vi "Configure 4Wire Resistance.vi"(0 "VISA resource name":refnum<visa-resource-name>, 1 "NPLC":u16(ring) items=["0.00005", "1", "12", "15"], 2 "Offset Compensation":bool, 5 "Auto Range? (T: Auto)":bool, 7 "Manual Range":dbl, 9 "Aperture Seconds":dbl, 11 "error in (no error)":errorcluster, 12 "Enable Dry Circuit":bool, 13 "Detection of Open Leads":bool) -> (4 "VISA resource name out":refnum<visa-resource-name>, 15 "error out":errorcluster)   [LabVIEW 2009, in "Keithley DMM7510.lvlib"]
doc: "This VI configures the 4 wire Resistance."
uses:
  Keithley DMM7510.lvlib
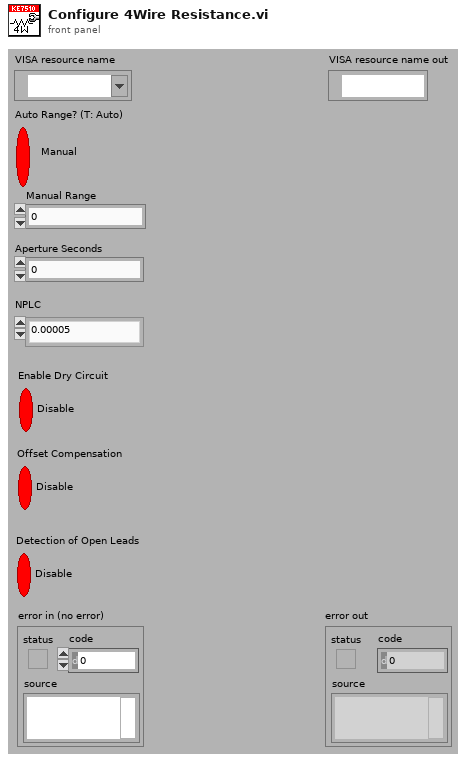
[diagram p1: front panel]
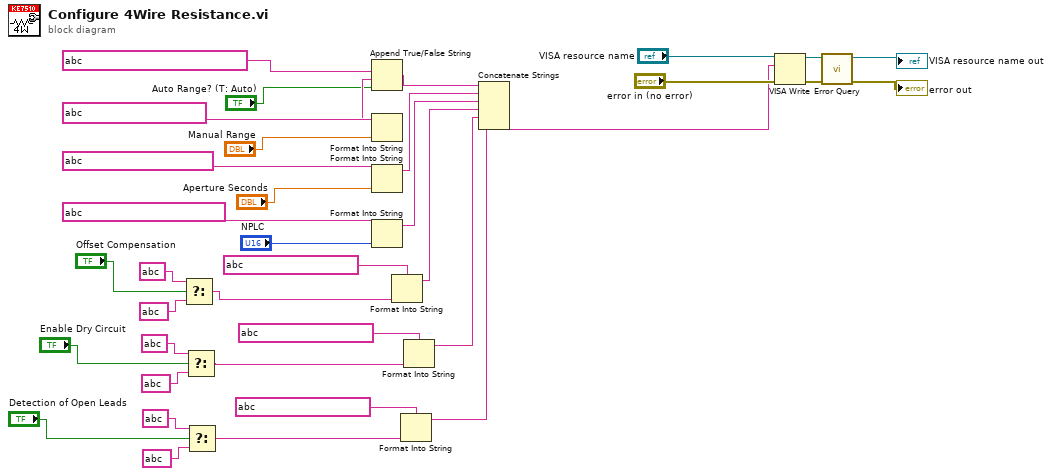
[diagram p0: block diagram]
diagram:
  n1 = Select(t=string ? ("format string"), s="Offset Compensation", f=string ? ("format string")) -> (s? t:f=w8:string)
  n2 = Select(t=string ? ("format string"), s="Enable Dry Circuit", f=string ? ("format string")) -> (s? t:f=w4:string)
  n3 = Select(t=string ? ("format string"), s="Detection of Open Leads", f=string ? ("format string")) -> (s? t:f=w7:string)
  n4 = Format Into String(format string=string ?, "Manual Range") -> (resulting string=w29:string)  [unwired: 2 in, 1 out]
  n5 = Append True/False String(1:"Auto Range? (T: Auto)", 2:w29, 3:string ?) -> (0:w26:string)  [unwired: 1 in]
  n6 = Format Into String(format string=string ?, "Aperture Seconds") -> (resulting string=w25:string)  [unwired: 2 in, 1 out]
  n7 = Format Into String(format string=string ?, "NPLC") -> (resulting string=w24:string)  [unwired: 2 in, 1 out]
  n8 = Format Into String(format string=string ?, w8) -> (resulting string=w3:string)  [unwired: 2 in, 1 out]
  n9 = Format Into String(format string=string ?, w7) -> (resulting string=w1:string)  [unwired: 2 in, 1 out]
  n10 = Format Into String(format string=string ?, w4) -> (resulting string=w2:string)  [unwired: 2 in, 1 out]
  n11 = Concatenate Strings(w26, w25, w24, w3, w2, w1) -> (w23:string)
  n12 = VISA Write(VISA resource name="VISA resource name", write buffer=w23, error in (no error)="error in (no error)") -> (VISA resource name out=w37:refnum<visa-resource-name>, error out=w36:errorcluster)  [unwired: 1 out]
  n13 = call "Error Query.vi"("error in (no error)"=w36, "VISA resource name"=w37) -> ("error out"=→"error out":errorcluster, "VISA resource name out"=→"VISA resource name out":refnum<visa-resource-name>)  [unwired: 6 in, 2 out]
